vi "Log Results.vi"(8 "error in (no error)":errorcluster, 10 "Mag Lab Result.lvclass":refnum<class "Mag Lab Result.lvclass">, 11 "Mag Lab Measure Controller in":refnum<class "Mag Lab Measure Controller.lvclass">) -> (0 "error out":errorcluster, 3 "Mag Lab Measure Controller out":refnum<class "Mag Lab Measure Controller.lvclass">)   [LabVIEW 2015, in "Mag Lab Measure Controller.lvclass"]
uses:
  Mag Lab Measure Controller.lvclass
  Mag Lab Result/Mag Lab Result.lvclass
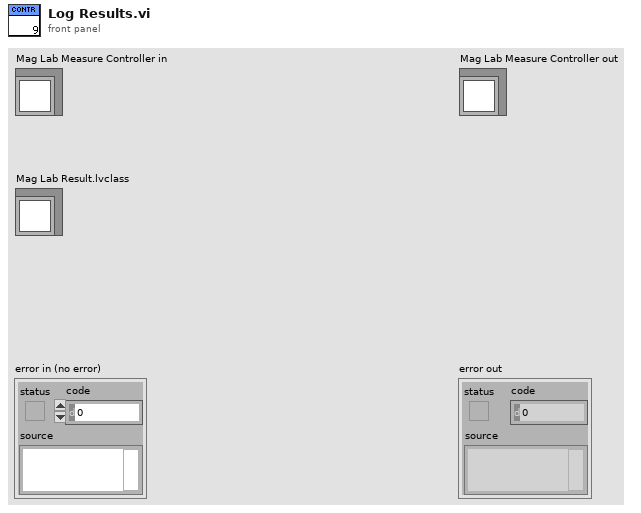
[diagram p1: front panel]
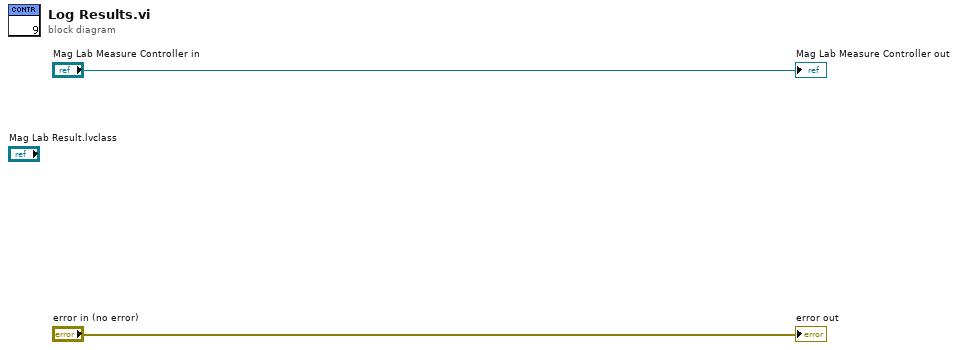
[diagram p0: block diagram]
diagram:
  "error out" <- "error in (no error)"
  "Mag Lab Measure Controller out" <- "Mag Lab Measure Controller in"
